vi "Read.vi"(4 "Error In":errorcluster, 7 "Plugin Name":T1) -> (0 "Error Out":errorcluster, 3 "Sample Period (msec)":i32)   [LabVIEW 2015, in "Sample Rate.lvlib"]
uses:
  Sample Rate.lvlib
  _libraries/Startup Processes/_typedefs/Subpanel Names.ctl
  _libraries/Startup Processes/Startup Processes.lvlib
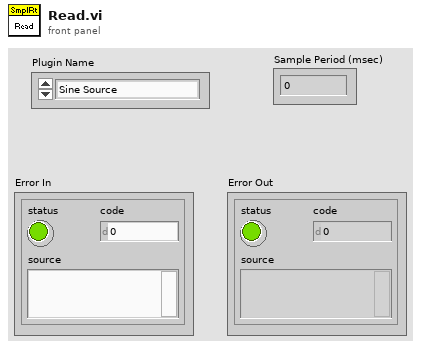
[diagram p1: front panel]
types:
  T1 = typedef "Startup Processes.lvlib/Subpanel Names.ctl" = enum16{"Sine Source", "Ramp Source", "Hen House TC", "Dog House TC", "Out House TC"}
  T2 = typedef "Sample Rate.lvlib/data.ctl" = cluster{"Sine Sample Period":i32, "Ramp Sample Period":i32}
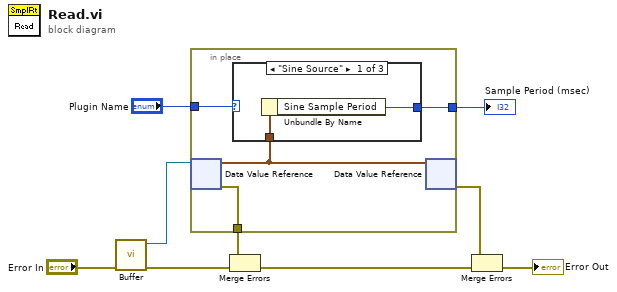
[diagram p0: block diagram]
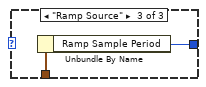
[diagram p3: hidden frame]
diagram:
  n1 = call "Buffer.vi"("Error In"="Error In") -> ("Error Out"=w5:errorcluster, "DVR"=w8:refnum<data-value>)  [unwired: 5 in]
  n2 = in-place {
    in-place-border: [w11] -> w7
    in-place-border: [w12] -> w4
    in-place-border: "Plugin Name" -> [w10]
    n3 = in-place-dvr #1(w8) -> (w13:T2, w12:errorcluster)
    n4 = case shown="\"Sine Source\"" w10 {
      tunnel: w13 -> [w15 _ w17]
      tunnel: [w14 _ w16] -> w11
      frame "Sine Source" {
        n5 = Unbundle By Name(w15) -> ("Sine Sample Period"=w14:i32)
      }
      frame Default {
      }
      frame "Ramp Source" {
        n6 = Unbundle By Name(w17) -> ("Ramp Sample Period"=w16:i32)
      }
    }
    n7 = in-place-dvr #1(w13) -> (w3:errorcluster)  [unwired: 1 out]
  }
  "Sample Period (msec)" <- w7
  n8 = Merge Errors(w4, w5) -> (w6:errorcluster)
  n9 = Merge Errors(w3, w6) -> (→"Error Out":errorcluster)
